vi "Lock Topic.vi"(6 "PublicationPolicy":refnum<class "IPublicationPolicy.lvclass">, 8 "error in (no error)":errorcluster, 9 "Return Error Transport":refnum<class "ITransport.lvclass">, 10 "Publisher ID":string, 11 "Topic in":refnum<class "Topic.lvclass">) -> (0 "error out":errorcluster, 3 "Topic out":refnum<class "Topic.lvclass">)   [LabVIEW 2017, in "Mediator.lvlib" / "Topic.lvclass"]
doc: "<License>\nCopyright © 2017 Composed Systems, LLC | All rights reserved\nwww.composed.io\n\nAuthor: Ethan Stern <ethan.stern@composed.io>\n\nThis software is provided \"AS IS\" WITHOUT WARRANTIES, either express or implied, AND IS FOR EDUCATIONAL PURPOSES ONLY.\n</License>"
uses:
  Topic.lvclass
  gpm_packages/@cs/transport/Source/ITransport/ITransport.lvclass
  IMediator/IPublicationPolicy/IPublicationPolicy.lvclass
  Topic.lvclass/Topic.ctl
  <vilib>/ErrorRing/Error Ring.xnode
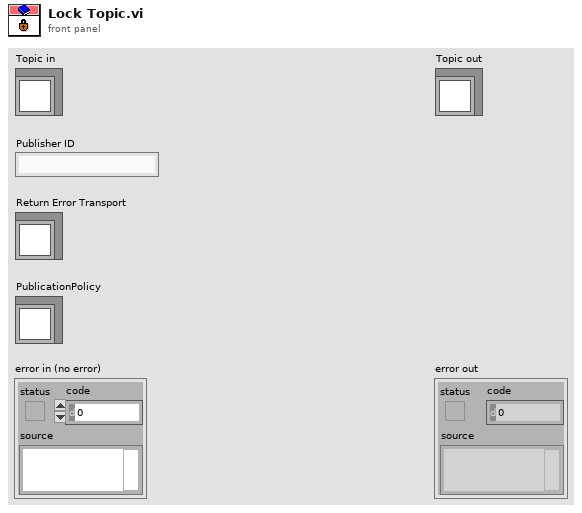
[diagram p1: front panel]
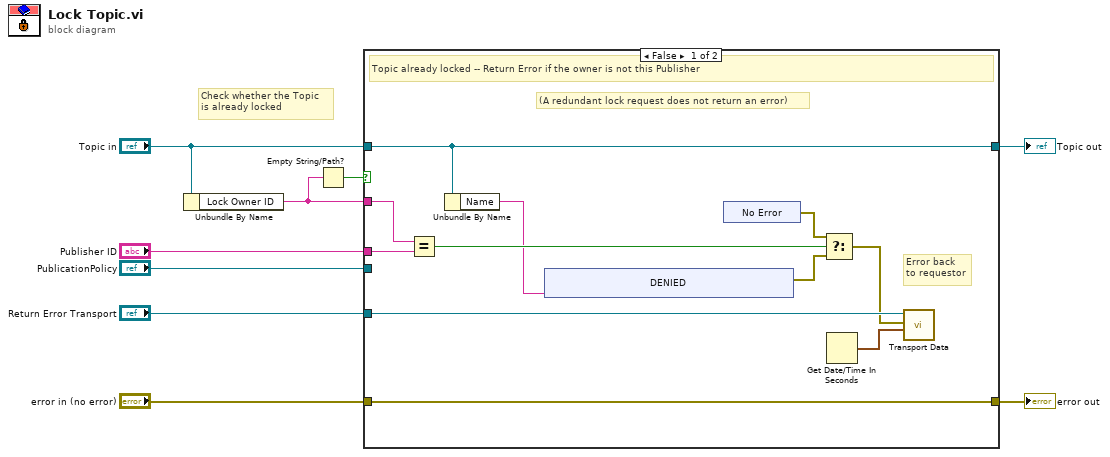
[diagram p0: block diagram]
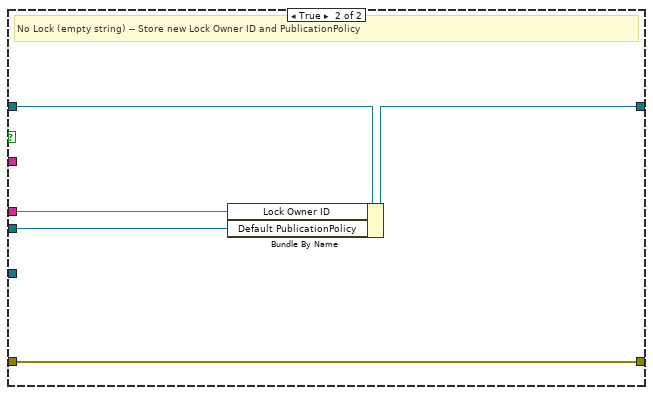
[diagram p2: hidden frame]
diagram:
  # "Check whether the Topic\nis already locked"
  n1 = Unbundle By Name("Topic in") -> ("Lock Owner ID"=w2:string)
  n2 = Empty String/Path?(string/path=w2) -> (empty?=w5:bool)
  n3 = case shown="False" w5 {
    tunnel: "error in (no error)" -> [w20 w28]
    tunnel: [w20 w28] -> w8
    tunnel: [w11 w30] -> w7
    tunnel: "Topic in" -> [w11 w31]
    tunnel: "Publisher ID" -> [w18 w29]
    tunnel: "Return Error Transport" -> [w14 _]
    tunnel: w2 -> [w19 _]
    tunnel: "PublicationPolicy" -> [_ w27]
    frame False {
      # "Error back\nto requestor"
      # "(A redundant lock request does not return an error)"
      # "Topic already locked -- Return Error if the owner is not this Publisher"
      n4 = Equal?(x=w19, y=w18) -> (x = y?=w17:bool)
      n5 = Unbundle By Name(w11) -> ("Name"=w10:string)
      n6 = xnode "DENIED"("parameter 0"=w10) -> ("error out"=w15:errorcluster)
      n7 = xnode "No Error"() -> ("error out"=w16:errorcluster)
      n8 = Select(t=w16, s=w17, f=w15) -> (s? t:f=w13:errorcluster)
      n9 = Get Date/Time In Seconds() -> (seconds since 1Jan1904=w12:timestamp)
      n10 = call "Transport Data.vi"("Publication Time (Get Time)"=w12, "Value"=w13, "ITransport in"=w14) -> ()  [unwired: 7 in, 2 out]
    }
    frame True {
      # "No Lock (empty string) -- Store new Lock Owner ID and PublicationPolicy"
      n11 = Bundle By Name(cluster=w31, "Lock Owner ID"=w29, "Default PublicationPolicy"=w27) -> (w30:refnum<class "Topic.lvclass">)
    }
  }
  "error out" <- w8
  "Topic out" <- w7
